vi "mqttCmdBuildVarHdr.vi"(0 "_mqtt in":refnum<class "BaseMqttMsg.lvclass">, 11 "error in (no error)":errorcluster) -> (4 "_mqtt out":refnum<class "BaseMqttMsg.lvclass">, 8 "variableHeader":u8[](array[numeric]) format="%02x", 15 "error out":errorcluster)   [LabVIEW 2020, in "BaseMqttMsg.lvclass"]
uses:
  BaseMqttMsg.lvclass
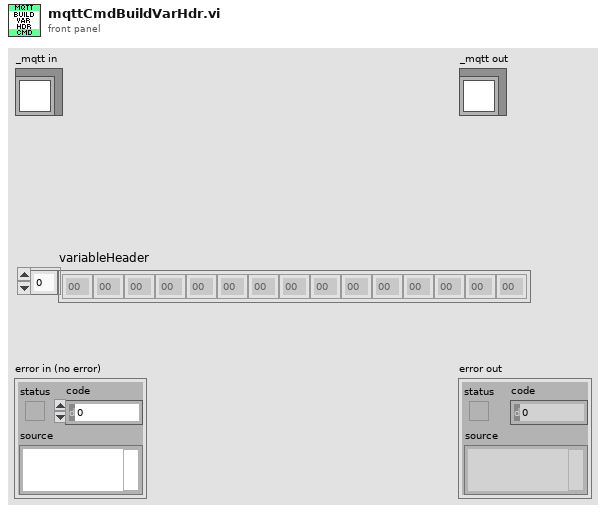
[diagram p1: front panel]
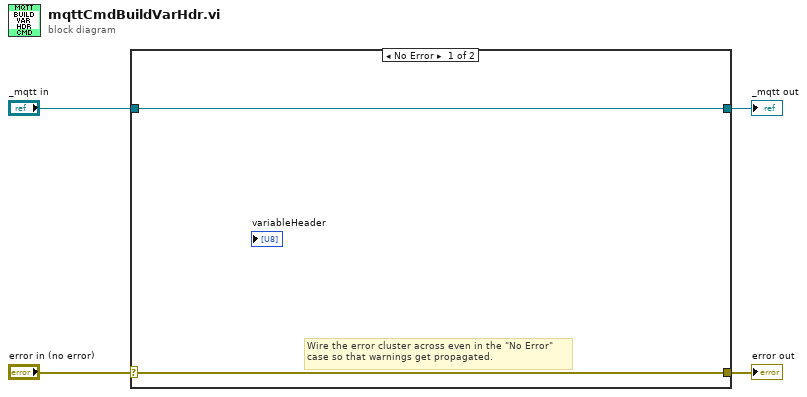
[diagram p0: block diagram]
diagram:
  n1 = case shown="No Error" "error in (no error)" {
    selector: "error in (no error)" -> [w5 w8]
    tunnel: [w5 w8] -> w3
    tunnel: [w6 w7] -> w1
    tunnel: "_mqtt in" -> [w6 w7]
    frame No Error {
      # "Wire the error cluster across even in the \"No Error\"\ncase so that warnings get propagated."
    }
    frame Error {
    }
  }
  "error out" <- w3
  "_mqtt out" <- w1
